vi "Read Mac Address.vi"(8 "error in (no error)":errorcluster, 11 "TrialBasedExperiment in":refnum<class "TrialBasedExperiment.lvclass">) -> (0 "error out":errorcluster, 2 "Mac Address":string, 3 "TrialBasedExperiment out":refnum<class "TrialBasedExperiment.lvclass">)   [LabVIEW 2010, in "TrialBasedExperiment.lvclass"]
uses:
  TrialBasedExperiment.lvclass
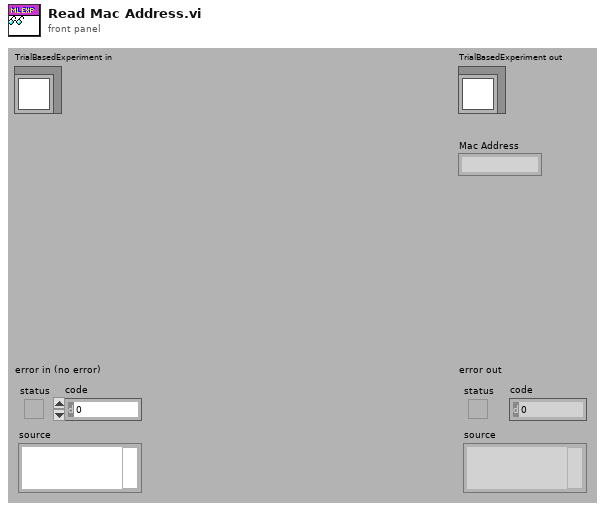
[diagram p1: front panel]
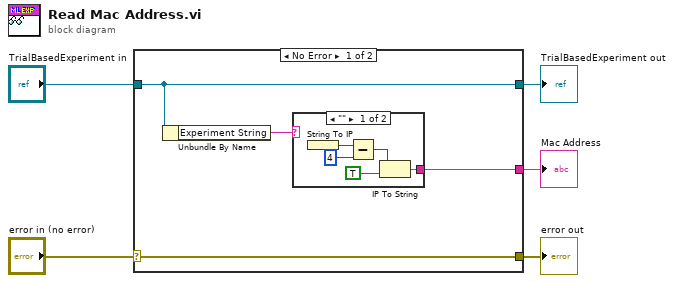
[diagram p0: block diagram]
diagram:
  n1 = case shown="No Error" "error in (no error)" {
    selector: "error in (no error)" -> [w9 w16]
    tunnel: [w9 w16] -> w4
    tunnel: [w8 w17] -> w2
    tunnel: "TrialBasedExperiment in" -> [w8 w17]
    tunnel: [w6 _] -> w1
    frame No Error {
      n2 = Unbundle By Name(w8) -> ("Experiment String"=w7:string)
      n3 = case shown="\"\"" w7 {
        selector: w7 -> [_ w15]
        tunnel: [w10 w15] -> w6
        frame "" {
          n4 = String To IP() -> (0:w14:u32)  [unwired: 1 out]
          n5 = Subtract(x=w14, y=u32 4) -> (x-y=w12:u32)
          n6 = IP To String(1:TRUE ("dot notation? (F)"), 2:w12) -> (0:w10:string)
        }
        frame "1", Default {
        }
      }
    }
    frame Error {
    }
  }
  "error out" <- w4
  "TrialBasedExperiment out" <- w2
  "Mac Address" <- w1
